vi "Main_Receiver.vi"(9 "Packet Parameters in":T2={"Length of sync sequence (50)"=50, "Number of message bits"=512, "Number of guardbits"=30, "Sync PN sequence order (31)"=31, "Number of header bits"=16, "Packet Pad [samples]"=200}, 10 "QPSK System Parameters":T4={"Samples per Symbol"=8, "symbol map"=[], "Differential PSK"=enum."enable", "PSK type"=0, "M-PSK"=4} {"PSK type" items=["normal", "shifted", "offset"]; "symbol map" format="%.3f"}) -> ()   [LabVIEW 2014]
uses:
  <vilib>/addons/Modulation/Digital/General/MT Generate Bits (Galois, PN Order).vi
  <vilib>/addons/Modulation/Digital/Support/Common/Validators/mod_Generate Bits Validate.vi
  <vilib>/addons/Modulation/Analog/support/mod_Set Error Source.vi
  <vilib>/addons/Modulation/Digital/General/subVIs/mod_Generate Bits PN Sequence.vi
  <instrlib>/niUSRP/niUSRP Fetch Rx Data (CDB Cluster).vi
  <vilib>/Analysis/NI_AALBase.lvlib
  <vilib>/addons/Modulation/niDMT.lvlib
panel:
  out "Packet loss [%]":dbl
  out "Eff. bit rate [bits/s]":dbl
  out "Packets lost":i32
  out "Bit error rate":dbl
  out "Data bits received":i32
  out "Bit errors":i32
  out "Sync Ok?":bool
  out "Packets Received":i32
  out "Waveform Graph":dbl[](graph)
  in  "Test Setup":T1={"Packets to send"=100, "Queue Length"=10, "PN sequence order (9)"=9}
  out "Symbol Rate [Hz]":dbl
  out "Median Sync Index":dbl format="%0.2f"
  out "Frame Length [samples]":i32
  in  "stop 2":bool
  out "Expected Sync Index":i32
  out "error out":errorcluster
  in  "error in (no error)":errorcluster
  in  "filter parameters":T3={"Alpha"=0.5, "Filter Length"=6, "TX Filter"=enum."Root Raised Cos"} {"Alpha" format="%.2f"}
  in  "USRP IP Address 2":refnum<k15>="192.168.10.1"
  out "Actual Rx Parameters  2":T5={"Rx IQ Sampling\nRate [s/sec]"=200000.0, "Rx\nFrequency [Hz]"=915000000.0, "Rx Gain [dB]"=20.0, "Rx Antenna"="RX1"} {"Rx Gain [dB]" format="%#.6p"; "Rx\nFrequency [Hz]" format="%#.6p"; "Rx IQ Sampling\nRate [s/sec]" format="%#.6p"}
  in  "Rx Parameters":T5={"Rx IQ Sampling\nRate [s/sec]"=400000.0, "Rx\nFrequency [Hz]"=2450000000.0, "Rx Gain [dB]"=20.0, "Rx Antenna"="RX1"} {"Rx Gain [dB]" format="%#.6p"; "Rx\nFrequency [Hz]" format="%#.6p"; "Rx IQ Sampling\nRate [s/sec]" format="%#.6p"}
  # "Calculated values"
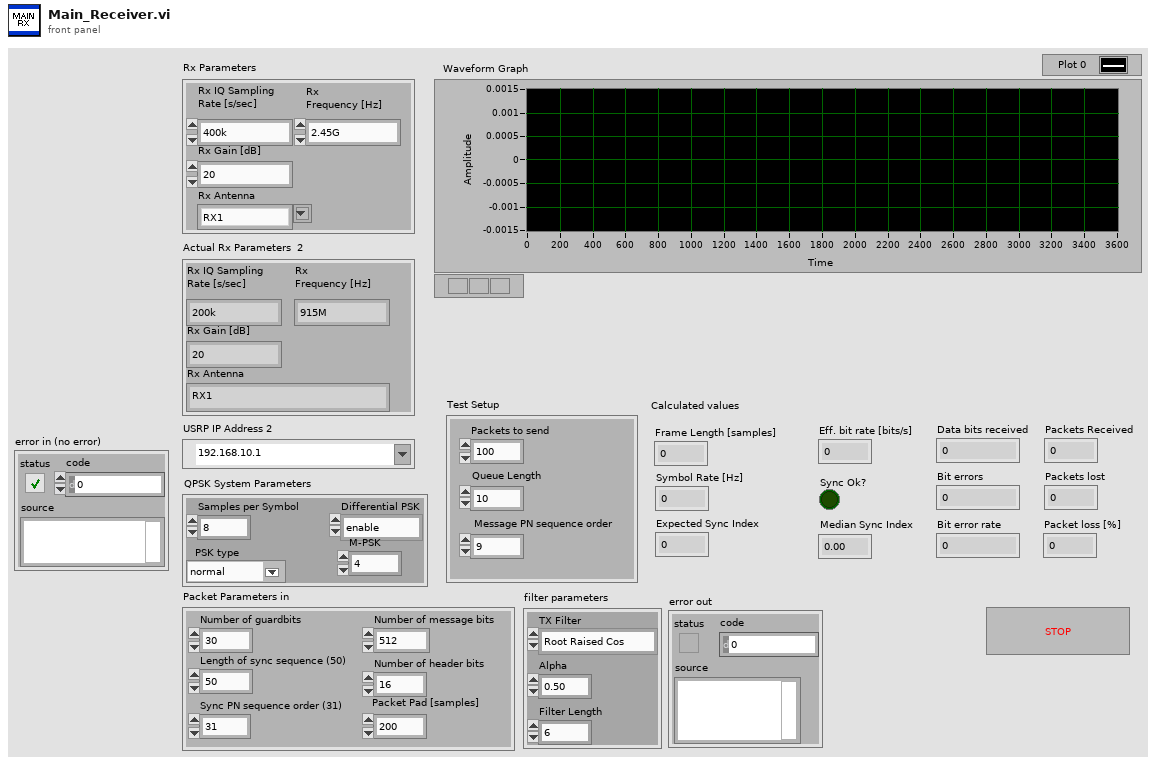
[diagram p1: front panel]
types:
  T1 = cluster{"Packets to send":i32, "Queue Length":i32, "PN sequence order (9)":i32}
  T2 = cluster{"Length of sync sequence (50)":i32, "Number of message bits":i32, "Number of guardbits":i32, "Sync PN sequence order (31)":i32, "Number of header bits":i32, "Packet Pad [samples]":i32}
  T3 = cluster{"Alpha":dbl, "Filter Length":i32, "TX Filter":enum16{"none", "Raised Cosine", "Root Raised Cos", "Gaussian"}}
  T4 = cluster{"Samples per Symbol":i32, "symbol map":cdb[], "Differential PSK":enum16{"disable", "enable"}, "PSK type":u16, "M-PSK":i32}
  T5 = cluster{"Rx IQ Sampling\nRate [s/sec]":dbl, "Rx\nFrequency [Hz]":dbl, "Rx Gain [dB]":dbl, "Rx Antenna":string}
  T6 = cluster{"samples per symbol (16)":i32, "symbol map":cdb[], "differential PSK":enum16{"disable", "enable"}, "PSK type":u16}
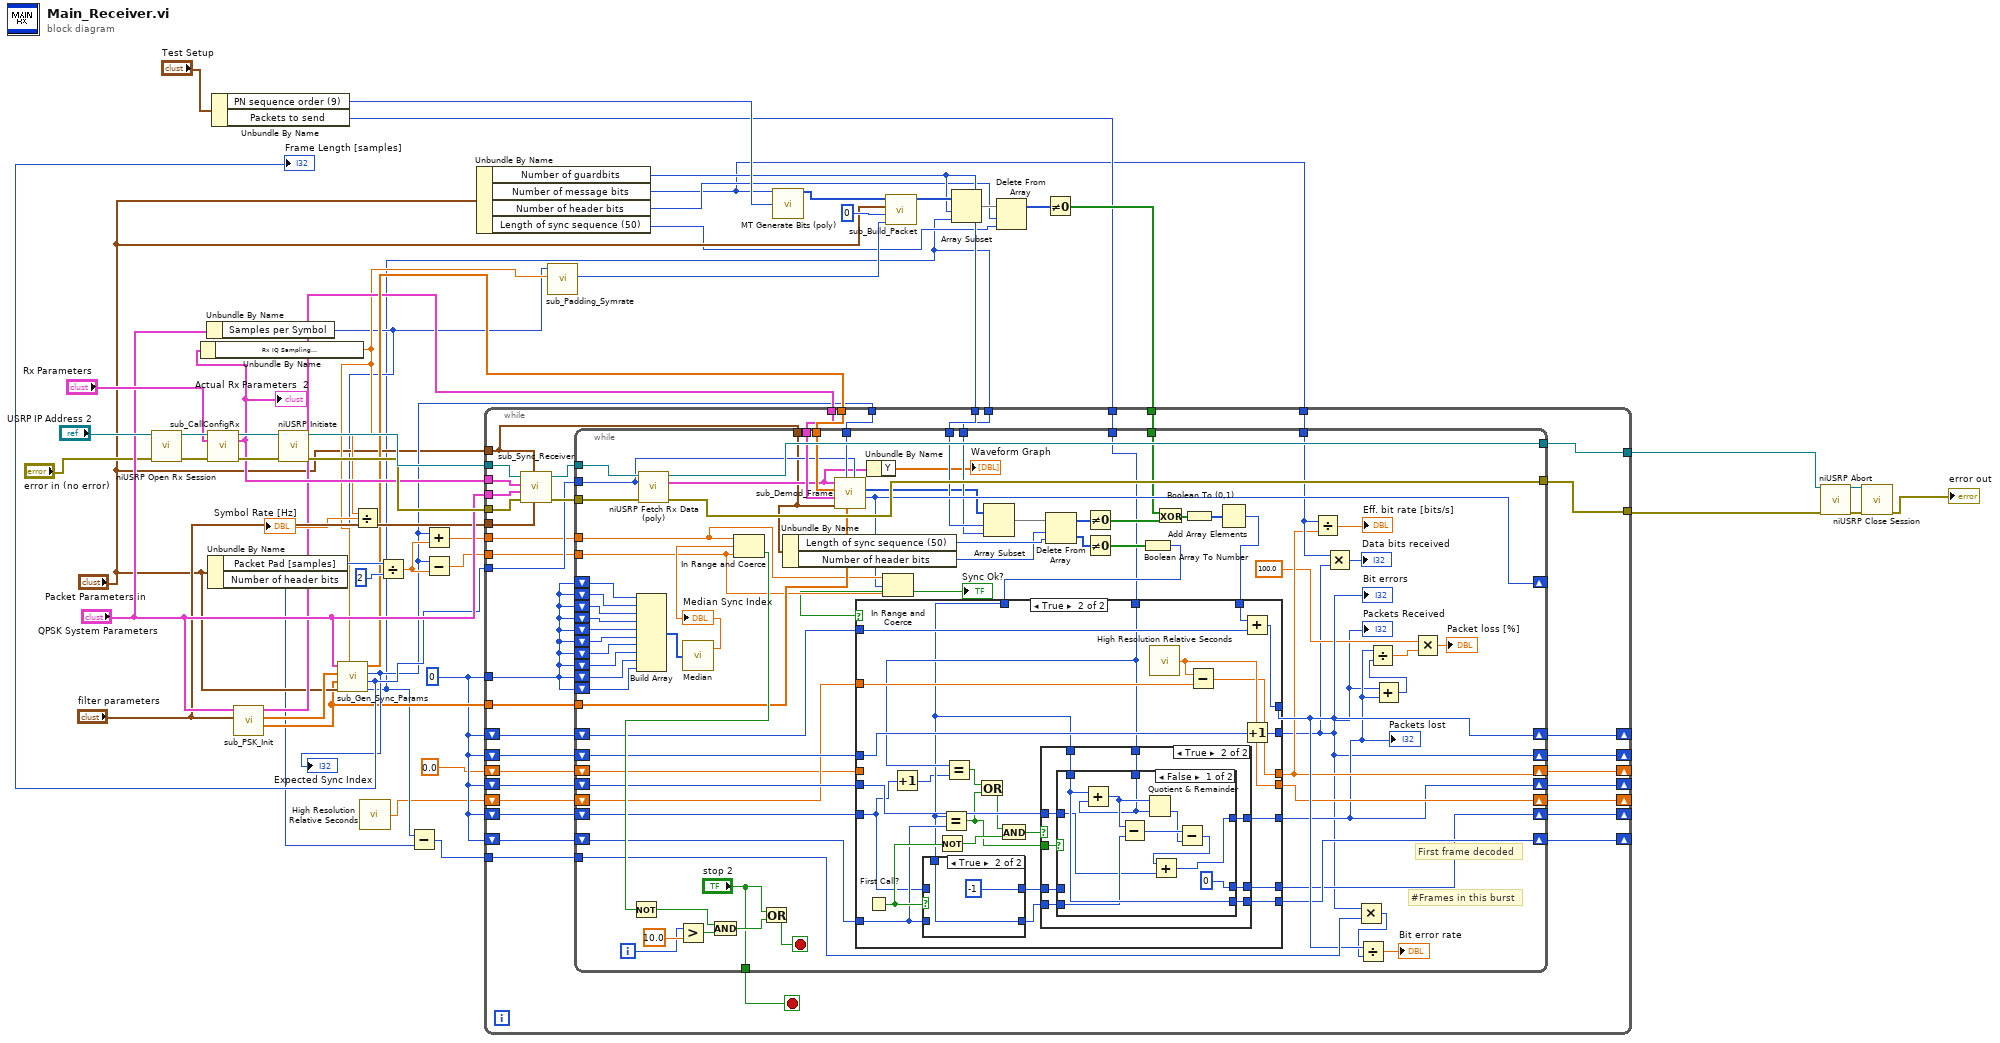
[diagram p0: block diagram]
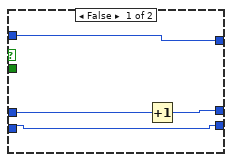
[diagram p3: hidden frame]
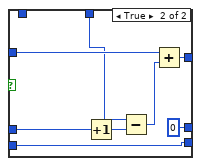
[diagram p4: hidden frame]
diagram:
  w8 = 0 ("y")
  n1 = call <instrlib>:"niUSRP Open Rx Session.vi"("device names"="USRP IP Address 2", "error in (no error)"="error in (no error)") -> ("session handle out"=w51:refnum<k15>, "error out"=w52:errorcluster)  [unwired: 12 in]
  n2 = Unbundle By Name("QPSK System Parameters") -> ("Samples per Symbol"=w13:i32)
  n3 = call "sub_CallConfigRx.vi"("session handle"=w51, "Rx Parameters"="Rx Parameters", "error in"=w52) -> ("session handle out"=w50:refnum<k15>, "Actual Rx Parameters"=w36:T5, "error out"=w49:errorcluster)  [unwired: 10 in]
  "Actual Rx Parameters  2" <- w36
  n4 = Unbundle By Name(w36) -> ("Rx IQ Sampling\nRate [s/sec]"=w16:dbl)
  n5 = Unbundle By Name("Packet Parameters in") -> ("Packet Pad [samples]"=w35:i32, "Number of header bits"=w5:i32)
  n6 = Unbundle By Name("Test Setup") -> ("PN sequence order (9)"=w28:i32, "Packets to send"=w4:i32)
  n7 = call "sub_PSK_Init.vi"("filter parameters in"="filter parameters", "QPSK System Parameters in"="QPSK System Parameters") -> ("matched filter coefficients"=w14:dbl[], "pulse shaping filter coefficients"=w23:dbl[], "PSK system parameters"=w21:T6)  [unwired: 7 in]
  n8 = call <instrlib>:"niUSRP Initiate.vi"("session handle"=w50, "error in (no error)"=w49) -> ("session handle out"=w47:refnum<k15>, "error out"=w46:errorcluster)  [unwired: 12 in]
  n9 = call "sub_Gen_Sync_Params.vi"("IQ Sampling\nRate [s/sec]"=w16, "Packet Parameters in"="Packet Parameters in", "matched filter coefficients"=w14, "pulse shaping filter coefficients"=w23, "QPSK System Parameters in"="QPSK System Parameters") -> ("Payload length"=w6:i32, "Frame Length (samples)"=w20:i32, "Expected Xcorr Index"=w19:i32, "Sync Sequence Waveform"=w22:cdb[])  [unwired: 3 in]
  "Expected Sync Index" <- w19
  "Frame Length [samples]" <- w20
  n10 = Divide(x=w16, y=w13) -> (x/y=→"Symbol Rate [Hz]":dbl)
  n11 = call <vilib>:"High Resolution Relative Seconds.vi"() -> ("relative seconds"=w2:dbl)
  n12 = Divide(x=w35, y=2) -> (x/y=w33:dbl)
  n13 = Subtract(x=w6, y=w5) -> (x-y=w7:i32)
  n14 = Add(x=w19, y=w33) -> (x+y=w32:dbl)
  n15 = Subtract(x=w19, y=w33) -> (x-y=w31:dbl)
  n16 = Unbundle By Name("Packet Parameters in") -> ("Number of guardbits"=w18:i32, "Number of message bits"=w3:i32, "Number of header bits"=w10:i32, "Length of sync sequence (50)"=w11:i32)
  n17 = call "sub_Padding_Symrate.vi"("Tx IQ Sampling\nRate [s/sec]"=w16, "Samples per Symbol"=w13) -> ("Padding Bits"=w25:i32)  [unwired: 8 in, 1 out]
  n18 = call-poly <vilib>:"MT Generate Bits (poly).vi"("total bits (128)"=w3, "PN sequence order (9)"=w28) -> ("output bit stream"=w27:i8[])  [unwired: 11 in, 2 out]
  n19 = call "sub_Build_Packet.vi"("Cyclic Padding Bits"=w25, "Packet number"=i16 0, "Packet Parameters in"="Packet Parameters in", "Input Message"=w27) -> ("Packet out"=w24:i8[])  [unwired: 7 in]
  n20 = Array Subset(array=w24, index=w18, length=w6) -> (w12:i8[])
  n21 = Delete From Array(array=w12, length=w10, index=w11) -> (array with subset deleted=w9:i8[])  [unwired: 1 out]
  n22 = Not Equal To 0?(x=w9) -> (x != 0?=w17:bool[])
  n23 = while {
    tunnel: w47 -> [w91]
    tunnel: w46 -> [w90]
    tunnel: w36 -> [w89]
    tunnel: "QPSK System Parameters" -> [w88]
    tunnel: "filter parameters" -> [w87]
    tunnel: w20 -> [w84]
    tunnel: w22 -> [w83]
    tunnel: [w82] -> w40
    tunnel: [w81] -> w38
    tunnel: "Packet Parameters in" -> [w74]
    tunnel: w8 -> [w80]
    tunnel: w32 -> [w79]
    tunnel: w31 -> [w78]
    tunnel: w14 -> [w77]
    tunnel: w19 -> [w76]
    tunnel: w21 -> [w75]
    shift-right: [w72] -> _
    shift-left: w8 -> [w73]
    tunnel: w18 -> [w71]
    tunnel: w6 -> [w70]
    tunnel: w17 -> [w69]
    shift-right: [w67] -> _
    shift-left: w8 -> [w68]
    tunnel: w7 -> [w66]
    shift-right: [w64] -> _
    shift-left: w8 -> [w65]
    shift-right: [w62] -> _
    shift-left: w8 -> [w63]
    shift-right: [w60] -> _
    shift-left: w8 -> [w61]
    tunnel: w4 -> [w59]
    tunnel: w3 -> [w58]
    shift-right: [w55] -> _
    shift-left: w2 -> [w57]
    shift-right: [w54] -> _
    shift-left: 0.0 -> [w56]
    stop <- w53 stop-if-true
    n24 = call "sub_Sync_Receiver.vi"("filter parameters"=w87, "Packet Parameters in"=w74, "error in (no error)"=w90, "QPSK System Parameters"=w88, "Rx Parameters"=w89, "session handle"=w91) -> ("error out"=w85:errorcluster, "session handle out"=w86:refnum<k15>)  [unwired: 4 in]
    n25 = while {
      tunnel: w86 -> [w167]
      tunnel: w85 -> [w166]
      tunnel: w84 -> [w142]
      tunnel: w83 -> [w145]
      tunnel: [w165] -> w82
      tunnel: [w164] -> w81
      shift-right: [w139] -> _
      shift-left: w80 -> [w163]
      shift-left: w80 -> [w162]
      shift-left: w80 -> [w161]
      shift-left: w80 -> [w160]
      shift-left: w80 -> [w159]
      shift-left: w80 -> [w158]
      shift-left: w80 -> [w157]
      shift-left: w80 -> [w156]
      shift-left: w80 -> [w155]
      shift-left: w80 -> [w154]
      tunnel: w79 -> [w140]
      tunnel: w78 -> [w141]
      tunnel: w77 -> [w146]
      tunnel: w76 -> [w143]
      tunnel: w75 -> [w144]
      tunnel: w74 -> [w121]
      shift-right: [w96] -> w72
      shift-left: w73 -> [w137]
      tunnel: w71 -> [w136]
      tunnel: w70 -> [w135]
      tunnel: w69 -> [w133]
      shift-right: [w127] -> w67
      shift-left: w68 -> [w129]
      tunnel: w66 -> [w128]
      shift-right: [w113] -> w64
      shift-left: w65 -> [w112]
      shift-right: [w111] -> w62
      shift-left: w63 -> [w110]
      shift-right: [w97] -> w60
      shift-left: w61 -> [w109]
      tunnel: w59 -> [w108]
      tunnel: w58 -> [w103]
      shift-right: [w104] -> w55
      shift-left: w57 -> [w106]
      shift-right: [w102] -> w54
      shift-left: w56 -> [w105]
      tunnel: ["stop 2"] -> w53
      i -> [w150]
      stop <- w94 stop-if-true
      # "First frame decoded"
      # "#Frames in this burst"
      n26 = Build Array(w163, w162, w161, w160, w159, w158, w157, w156, w155, w154) -> (w153:i32[])
      n27 = call-poly <instrlib>:"niUSRP Fetch Rx Data (poly).vi"("session handle"=w167, "number of samples"=w142, "error in (no error)"=w166) -> ("session handle out"=w164:refnum<k15>, "data"=w123:cluster{"t0":dbl, "dt":dbl, "Y":cdb[]}, "error out"=w165:errorcluster)  [unwired: 9 in, 1 out]
      n28 = Greater?(x=w150, y=10.0) -> (0:w149:bool)
      n29 = call <vilib>:"Median.vi"("X"=w153) -> ("median"=w152:dbl)  [unwired: 1 out]
      "Median Sync Index" <- w152
      n30 = In Range and Coerce(upper limit=w140, x=w152, lower limit=w141) -> (In Range?=w148:bool)  [unwired: 1 out]
      n31 = Not(x=w148) -> (.not. x?=w147:bool)
      n32 = And(x=w147, y=w149) -> (x .and. y?=w93:bool)
      n33 = Or(x="stop 2", y=w93) -> (x .or. y?=w94:bool)
      n34 = Unbundle By Name(w121) -> ("Length of sync sequence (50)"=w116:i32, "Number of header bits"=w115:i32)
      n35 = call "sub_Demod_Frame.vi"("Packet Length [samples]"=w142, "matched filter coefficients"=w146, "Expected Xcorr Index"=w143, "Packet Parameters in"=w121, "PSK system parameters"=w144, "Sync Sequence Waveform"=w145, "Input Complex Waveform"=w123) -> ("Max Xcorr Index"=w139:i32, "output bit stream"=w122:i8[])  [unwired: 2 in, 1 out]
      n36 = Unbundle By Name(w123) -> ("Y"=→"Waveform Graph":cdb[])
      n37 = In Range and Coerce(upper limit=w140, x=w139, lower limit=w141) -> (In Range?=w138:bool)  [unwired: 1 out]
      "Sync Ok?" <- w138
      n38 = Array Subset(array=w122, index=w136, length=w135) -> (w118:i8[])
      n39 = Delete From Array(array=w118, length=w115, index=w116) -> (deleted portion=w117:i8[], array with subset deleted=w119:i8[])
      n40 = Not Equal To 0?(x=w119) -> (x != 0?=w134:bool[])
      n41 = Not Equal To 0?(x=w117) -> (x != 0?=w120:bool[])
      n42 = Boolean Array To Number(Boolean array=w120) -> (number=w114:u32)
      n43 = Exclusive Or(1:w134, 2:w133) -> (0:w132:bool[])
      n44 = Boolean To (0,1)(Boolean=w132) -> (0, 1=w131:i16[])
      n45 = Add Array Elements(numeric array=w131) -> (sum=w130:i16)
      n46 = case shown="True" w138 {
        tunnel: w137 -> [w174 w199]
        tunnel: [w174 w198] -> w96
        tunnel: w130 -> [_ w197]
        tunnel: [w173 w196] -> w127
        tunnel: w129 -> [w173 w195]
        tunnel: w114 -> [_ w179]
        tunnel: [w172 w178] -> w113
        tunnel: w112 -> [w172 w193]
        tunnel: [w171 w190] -> w111
        tunnel: w110 -> [w171 w176]
        tunnel: w109 -> [w170 w189]
        tunnel: w108 -> [_ w183]
        tunnel: [w170 w188] -> w97
        tunnel: w106 -> [w169 w185]
        tunnel: w105 -> [w168 _]
        tunnel: [w169 w186] -> w104
        tunnel: [w168 w184] -> w102
        frame False {
        }
        frame True {
          n47 = First Call?() -> (First Call?: T/F=w194:bool)
          n48 = Increment(x=w176) -> (x+1=w175:i32)
          n49 = case shown="True" w194 {
            tunnel: [w232 w234] -> w177
            tunnel: w179 -> [_ w234]
            tunnel: w193 -> [w232 _]
            tunnel: [w231 -1 ("y")] -> w187
            tunnel: w176 -> [w231 _]
            frame False {
            }
            frame True {
            }
          }
          n50 = Not(x=w194) -> (.not. x?=w192:bool)
          n51 = Equal?(x=w179, y=w193) -> (x = y?=w180:bool)
          n52 = Equal?(x=w183, y=w175) -> (x = y?=w182:bool)
          n53 = Or(x=w182, y=w180) -> (x .or. y?=w181:bool)
          n54 = And(x=w181, y=w192) -> (x .and. y?=w191:bool)
          n55 = case shown="True" w191 {
            tunnel: [w202 w212] -> w190
            tunnel: w187 -> [w203 w208]
            tunnel: w189 -> [w201 w211]
            tunnel: w183 -> [_ w210]
            tunnel: [w201 w209] -> w188
            tunnel: w180 -> [_ w207]
            tunnel: w179 -> [_ w206]
            tunnel: [w200 w204] -> w178
            tunnel: w177 -> [w200 w205]
            frame False {
              n56 = Increment(x=w203) -> (x+1=w202:i32)
            }
            frame True {
              n57 = case shown="False" w207 {
                tunnel: [0 ("y") 0 ("y")] -> w212
                tunnel: w211 -> [w215 w228]
                tunnel: w210 -> [w218 w227]
                tunnel: [w213 w226] -> w209
                tunnel: w208 -> [_ w224]
                tunnel: w206 -> [w221 _]
                tunnel: w205 -> [w220 w223]
                tunnel: [w221 w223] -> w204
                frame False {
                  n58 = Add(x=w221, y=w218) -> (x+y=w219:u32)
                  n59 = Subtract(x=w219, y=w220) -> (x-y=w217:u32)
                  n60 = Quotient & Remainder(x=w219, y=w218) -> (floor(x/y)=w216:u32)  [unwired: 1 out]
                  n61 = Subtract(x=w217, y=w216) -> (x-y=w214:u32)
                  n62 = Add(x=w214, y=w215) -> (x+y=w213:u32)
                }
                frame True {
                  n63 = Increment(x=w224) -> (x+1=w225:i32)
                  n64 = Subtract(x=w227, y=w225) -> (x-y=w229:i32)
                  n65 = Add(x=w228, y=w229) -> (x+y=w226:u32)
                }
              }
            }
          }
          n66 = call <vilib>:"High Resolution Relative Seconds.vi"() -> ("relative seconds"=w186:dbl)
          n67 = Subtract(x=w186, y=w185) -> (x-y=w184:dbl)
          n68 = Add(x=w197, y=w195) -> (x+y=w196:i32)
          n69 = Increment(x=w199) -> (x+1=w198:i32)
        }
      }
      "Packets Received" <- w96
      "Bit errors" <- w127
      "Packets lost" <- w97
      n70 = Divide(x=w103, y=w102) -> (x/y=→"Eff. bit rate [bits/s]":dbl)
      n71 = Multiply(x=w103, y=w96) -> (x*y=→"Data bits received":i32)
      n72 = Multiply(x=w96, y=w128) -> (x*y=w126:i32)
      n73 = Divide(x=w127, y=w126) -> (x/y=→"Bit error rate":dbl)
      n74 = Add(x=w96, y=w97) -> (x+y=w95:u32)
      n75 = Divide(x=w97, y=w95) -> (x/y=w100:dbl)
      n76 = Multiply(x=100.0, y=w100) -> (x*y=→"Packet loss [%]":dbl)
    }
  }
  n77 = call <instrlib>:"niUSRP Abort.vi"("session handle"=w38, "error in (no error)"=w40) -> ("session handle out"=w41:refnum<k15>, "error out"=w42:errorcluster)  [unwired: 12 in]
  n78 = call <instrlib>:"niUSRP Close Session.vi"("session handle"=w41, "error in (no error)"=w42) -> ("error out"=→"error out":errorcluster)  [unwired: 13 in]
